vi "Parse Timestamp Array.vi"(6 "Seperator":string=",", 8 "error in":errorcluster, 9 "Input <JSON>":string, 10 "csv string":string, 11 "IParse CSV in":refnum<class "IParse CSV.lvclass">) -> (0 "error out":errorcluster, 2 "Timestamp Array":timestamp[](array[timestamp]) format="%<%x %.3X>T", 3 "IParse CSV out":refnum<class "IParse CSV.lvclass">)   [LabVIEW 2024, in "IParse CSV.lvclass"]
uses:
  IParse CSV.lvclass
  caab95f8-5789-4ddc-a871-2f845017f8a1.vi
  614d4d88-d356-4e27-8790-84129eebb769.vi
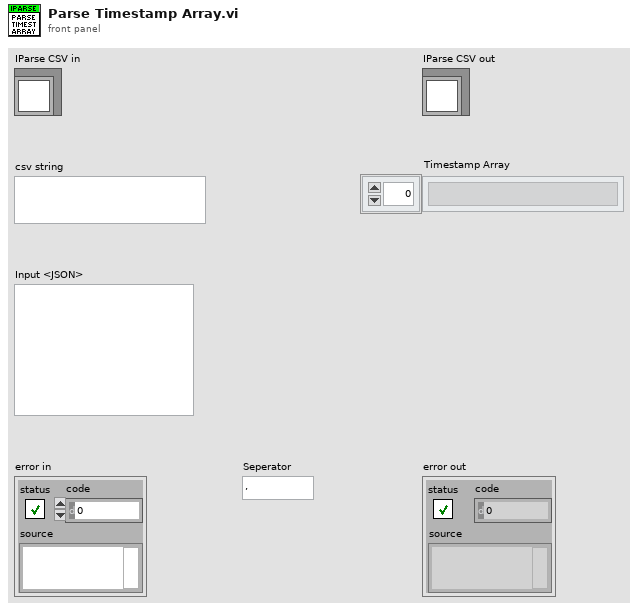
[diagram p1: front panel]
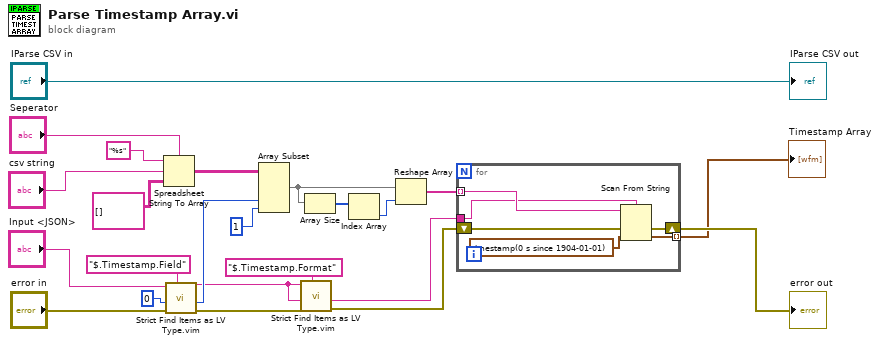
[diagram p0: block diagram]
diagram:
  n1 = Spreadsheet String To Array(delimiter (Tab)="Seperator", format string="%s", spreadsheet string="csv string", array type (2D Dbl)=string[][] []) -> (array=w19:string[][])
  n2 = call "Strict Find Items as LV Type.vim"("$Path or Item Name"="$.Timestamp.Field", "error in"="error in", "Data Type and Default Value"=0, "<JSON>"="Input <JSON>") -> ("error out"=w5:errorcluster, "Data out"=w6:i32, "<JSON> dup"=w2:string)  [unwired: 5 in]
  n3 = Array Subset(array=w19, index (col)=w6, length (col)=1 ("length")) -> (w17:string[][])  [unwired: 2 in]
  n4 = call "Strict Find Items as LV Type.vim"("$Path or Item Name"="$.Timestamp.Format", "error in"=w5, "Data Type and Default Value"=w2, "<JSON>"=w2) -> ("error out"=w4:errorcluster, "Data out"=w1:string)  [unwired: 5 in, 1 out]
  n5 = Array Size(array=w17) -> (size(s)=w18:i32[])
  n6 = Index Array(array=w18) -> (element=w16:i32)  [unwired: 1 in]
  n7 = Reshape Array(w17, w16) -> (w13:string[])
  n8 = for {
    shift-right: [w28] -> w14
    shift-left: w4 -> [w29]
    tunnel: w13 -> [w27] mode=indexing
    tunnel: [w26] -> w12 mode=indexing
    tunnel: w1 -> [w24]
    n9 = Scan From String(format string=w24, input string=w27, error in=w29, default 1=timestamp(0 s since 1904-01-01) ("Time Stamp")) -> (error out=w28:errorcluster, output 1=w26:timestamp)  [unwired: 1 in, 2 out]
  }
  "error out" <- w14
  "Timestamp Array" <- w12
  "IParse CSV out" <- "IParse CSV in"
